vi "Divide.vi"   [LabVIEW 2016, in "xy_utilities.lvlib"]
uses:
  xy_utilities.lvlib
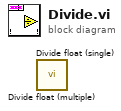
[diagram p0: block diagram]
diagram:
  n1 = call "Divide float (multiple).vi"() -> ()  [unwired: 10 in, 2 out]
  n2 = call "Divide float (single).vi"() -> ()  [unwired: 10 in, 2 out]
